vi "algoritmo_9.vi"() -> ()   [LabVIEW 2024]
uses:
  <vilib>/Platform/TimedLoop/XDataNode/timing_clust.ctl
  <vilib>/Platform/TimedLoop/XDataNode/nitl_modes.ctl
  <vilib>/Platform/TimedLoop/XDataNode/wakeup.ctl
  <vilib>/MakerHub/LINX/Public/Peripherals/PWM/PWM Set Duty Cycle 1 Chan.vi
  <vilib>/MakerHub/LINX/Public/Utilities/Open Serial.vi
  <vilib>/MakerHub/LINX/Public/Peripherals/PWM/PWM Set Duty Cycle N Chans.vi
  <vilib>/platform/TimedLoop/XDataNode/XDataNode.xnode
  <vilib>/Platform/TimedLoop/XDataNode/XDNodeRunTimeDep.lvlib
  <vilib>/MakerHub/LINX/LMH-LINX.lvlib
  <vilib>/MakerHub/LINX/Public/Sensors/Distance/Ultrasonic/Ultrasonic.lvlib
  <vilib>/Analysis/NI_AALPro.lvlib
panel:
  out "normal":dbl
  out "Integral":dbl
  out "poli":dbl
  out "pol":dbl
  in  "ESTIMAR":dbl(slide) scale=-41.0..41.0
  in  "Ref":dbl(slide) scale=5.0..41.0
  in  "POL":dbl(slide) scale=0.5..0.9
  in  "POLI":dbl(slide) scale=0.0..0.1
  in  "CONTROL":dbl
  out "Error":dbl
  out "PWM":dbl format="%0.2f"
  out "uk":dbl
  out "ESTADO":dbl
  out "MINUTOS":dbl format="%#_2g"
  out "Y_e":dbl
  out "error de estimacion":dbl
  out "THETA":cdb[](array[numeric])
  out "Waveform Chart":T1(graph)
  in  "stop":bool
  in  "Serial Port":refnum<visa-resource-name>="N/A"
  out "Error Out":errorcluster
  out "Y_Real":fxp<+/-,64,32>
  # "0 PARA ESTIMAR\n1 PARA CONTROLAR"
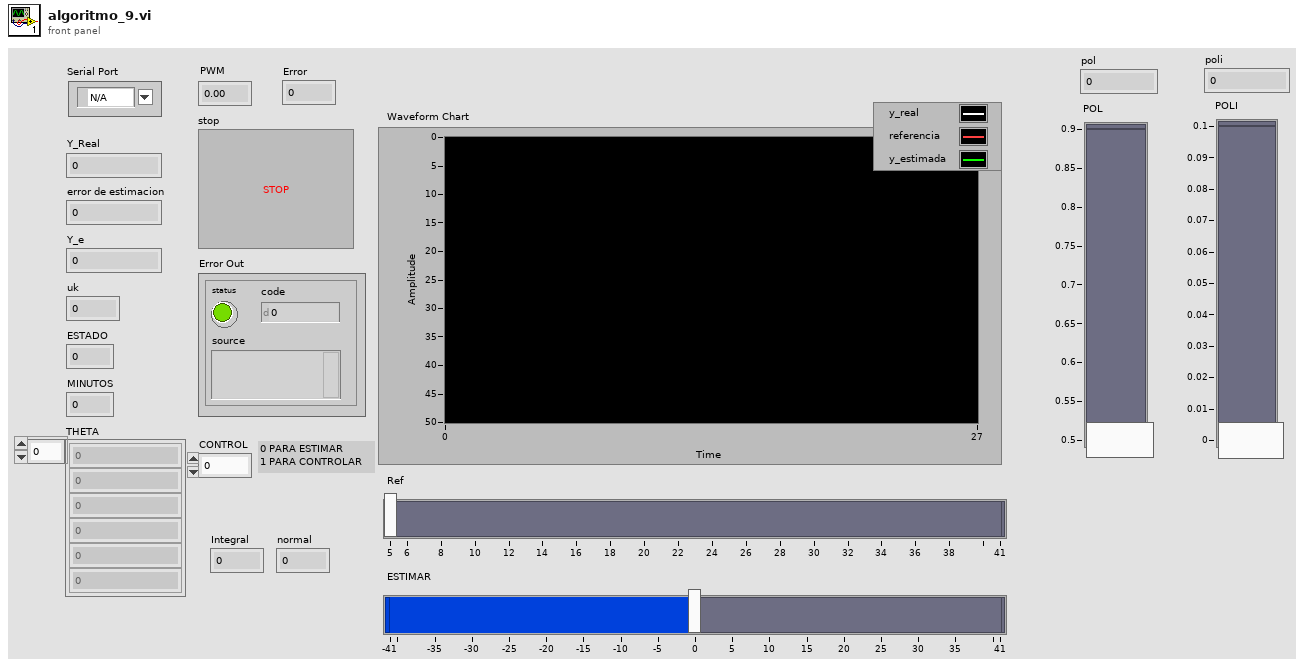
[diagram p1: front panel]
types:
  T1 = cluster{"Centimeters":dbl, "Referencia":dbl, dbl}
  T2 = typedef "LMH-LINX.lvlib/LINX Ref.ctl" = cluster{"IO":T3, "Interface":T4, "LINX Device Config":T5}
  T3 = typedef "LMH-LINX.lvlib/Platform.ctl" = enum16{"Remote", "Local"}
  T4 = typedef "LMH-LINX.lvlib/Interface.ctl" = enum16{"Serial", "TCP"}
  T5 = typedef "LMH-LINX.lvlib/Device.lvlib/LINX Device Config.ctl" = cluster{"Interface":T4, "COM Port":refnum<visa-resource-name>, "TCP Configuration":T6, "Device Family":u8, "Device ID":u8, "Device Name":string, "TCP Ref":refnum<k5>, "Channels":T7}
  T6 = typedef "LMH-LINX.lvlib/Device.lvlib/TCP Config.ctl" = cluster{"IP Address":string, "Port":u16}
  T7 = typedef "LMH-LINX.lvlib/Channels.ctl" = cluster{"DI":u8[], "DO":u8[], "AI":u8[], "AO":u8[], "PWM":u8[], "QE":u8[], "UART":u8[], "I2C 2":u8[], "SPI":u8[], "CAN":u8[], "Servo":u8[], "AI Ref (V)":dbl, "AI Resolution (Bits)":u8, "AO Ref (V)":dbl, "AO Resolution (Bits)":u8}
  T8 = typedef "XDNodeRunTimeDep.lvlib/timing_clust.ctl" = cluster{"Expected End [f-1]":u64, "Actual End [f-1]":u64, "Finished Late? [f-1]":bool, "Expected End [i-1]":u64, "Actual End [i-1]":u64, "Finished Late? [i-1]":bool, "Expected Start [i]":u64, "Actual Start [i]":u64, "Expected Start [f]":u64, "Actual Start [f]":u64, "Source Name":string, "Structure Name":string, "Period":i64, "Deadline":i64, "Offset":i64, "Start":i64, "Priority":i32, "Timeout":i32, "Mode":T9, "Wakeup Reason":T10, "Error":errorcluster, "Source Type":string, "Secondary Source Type":string, "Global End Time":u64, "Global Start Time":u64, "Frame Duration":u64, "Iteration Duration":u64, "Assigned CPU":i32, "I/O Scan Engine Mode":u32}
  T9 = typedef "XDNodeRunTimeDep.lvlib/nitl_modes.ctl" = enum32{"No Change", "Process missed periods, maintain original phase", "Discard missed periods, maintain original phase", "Process missed periods, ignore original phase", "Discard missed periods, ignore original phase"}
  T10 = typedef "XDNodeRunTimeDep.lvlib/wakeup.ctl" = enum32{"Normal", "Aborted", "Asynchronous wakeup", "Timing source error", "Timed loop error", "Timeout"}
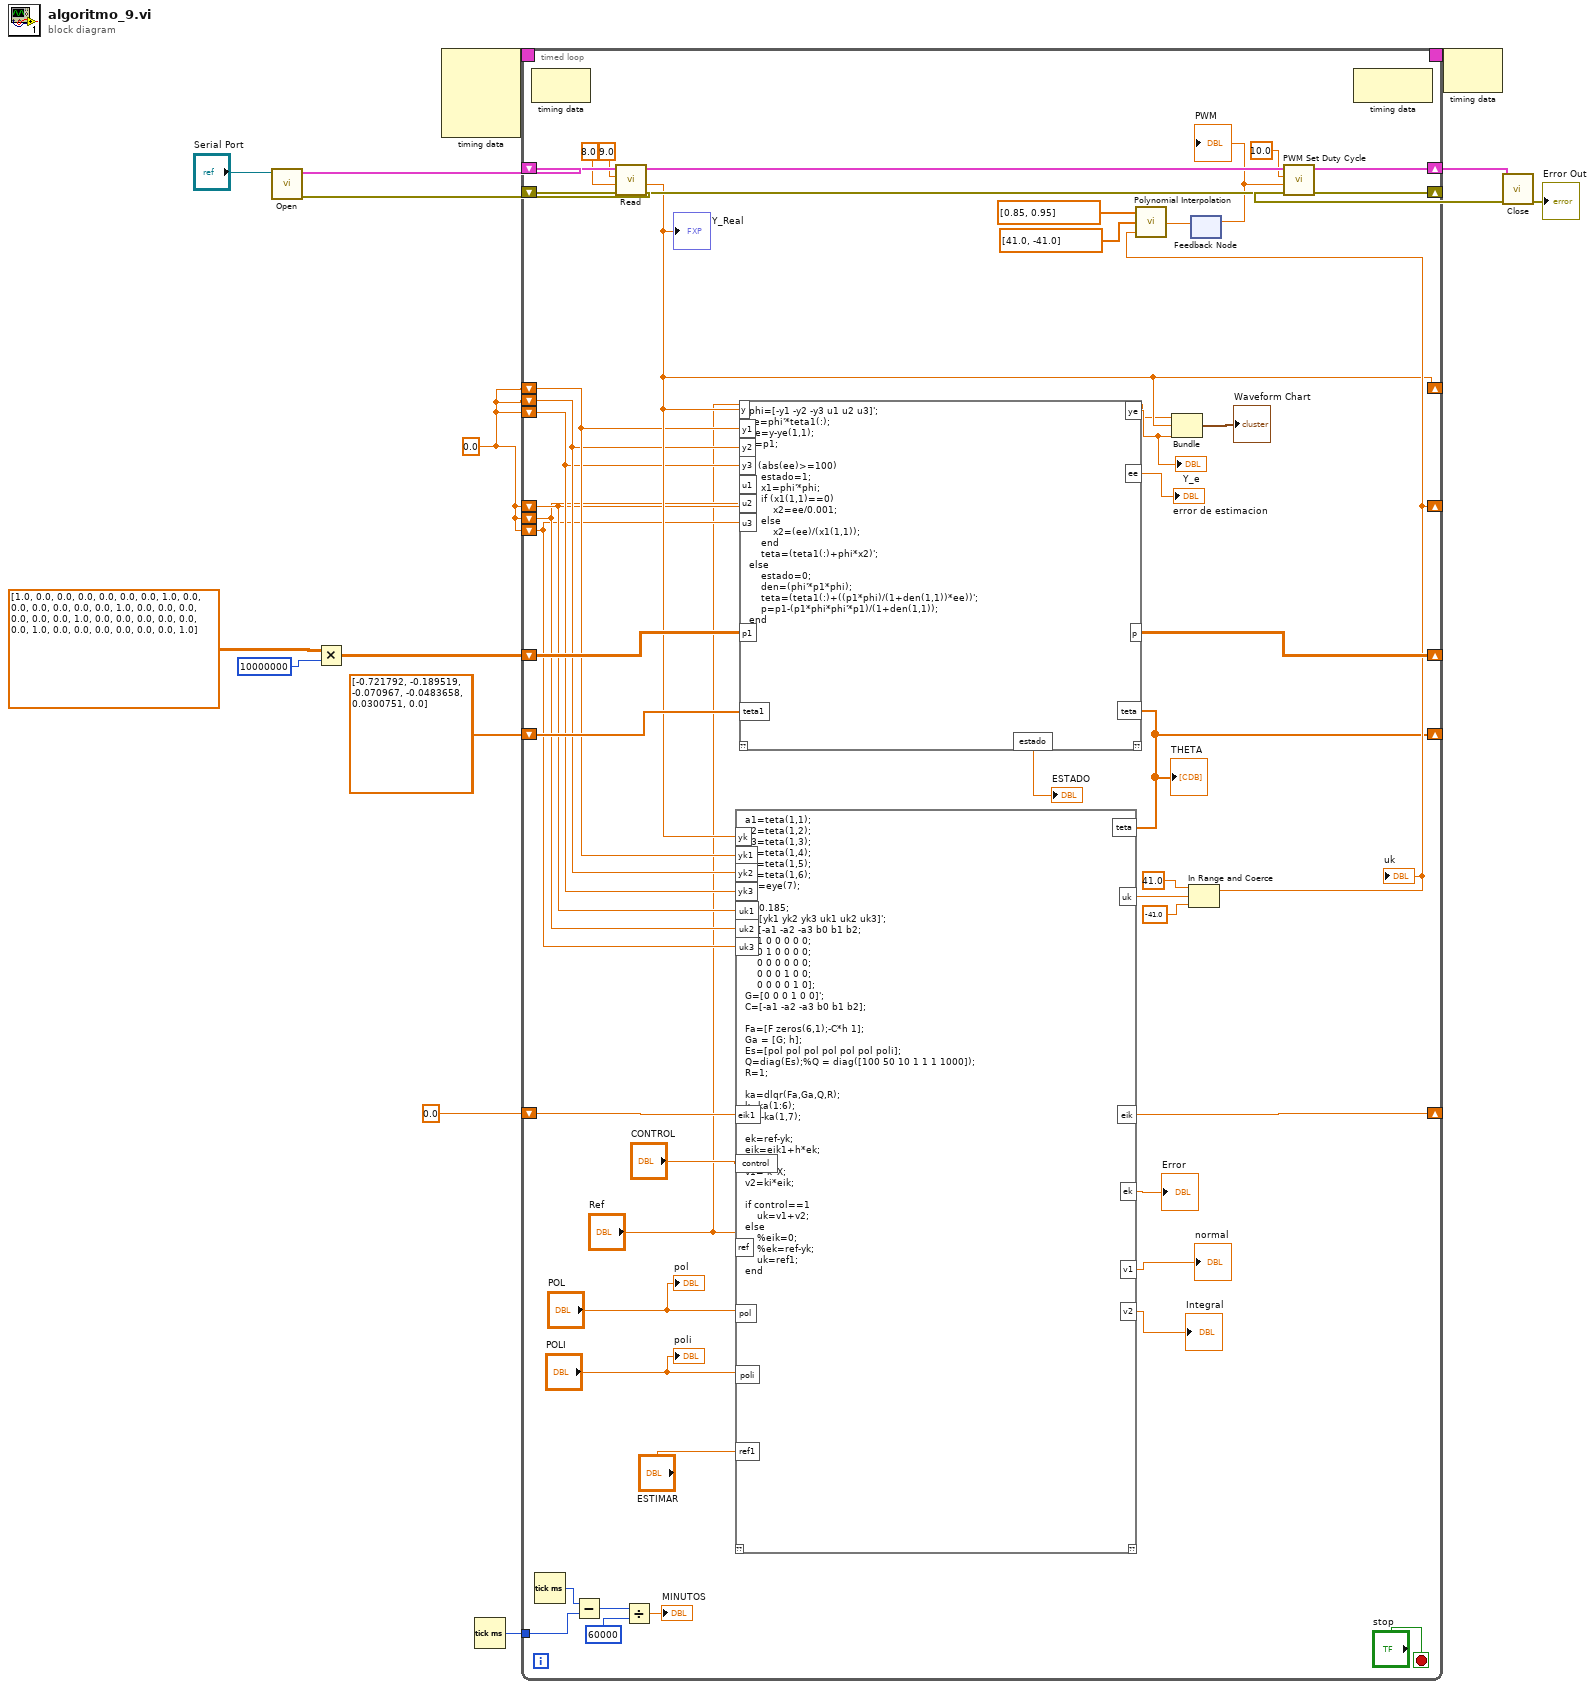
[diagram p0: block diagram]
diagram:
  (unwired) dbl[] [-0.721792, -0.189519, -0.070967, -0.0483658, 0.0300751, 0.0]
  w1 = 0.0
  n1 = call-poly <vilib>:"Open.vi"("Serial Port"="Serial Port") -> ("Error Out"=w11:errorcluster, "LINX Resource"=w13:T2)  [unwired: 8 in, 1 out]
  n2 = Multiply(x=dbl[][] [[1.0, 0.0, 0.0, 0.0, 0.0, 0.0], [0.0, 1.0, 0.0, 0.0, 0.0, 0.0], [0.0, 0.0, 1.0, 0.0, 0.0, 0.0], [0.0, 0.0, 0.0, 1.0, 0.0, 0.0], [0.0, 0.0, 0.0, 0.0, 1.0, 0.0], [0.0, 0.0, 0.0, 0.0, 0.0, 1.0]], y=10000000) -> (x*y=w5:dbl[][])
  n3 = node-c288() -> (w15:T8)  [unwired: 4 in]
  n4 = Tick Count (ms)() -> (millisecond timer value=w4:u32)
  n5 = timed-loop {
    timing: w15 -> [_]
    timing-out: [_] -> w14
    shift-right: [w52] -> w12
    shift-left: w13 -> [w63]
    shift-right: [w57] -> w10
    shift-left: w11 -> [w62]
    shift-right: [w23] -> _
    shift-left: dbl[] [-0.94337, -0.103907, 0.033856, -0.0056629, 0.00349643, 0.0144388] -> [w51]
    shift-right: [w30] -> _
    shift-left: w1 -> [w29]
    shift-right: [w31] -> _
    shift-left: w1 -> [w26]
    shift-left: w1 -> [w28]
    shift-left: w1 -> [w27]
    shift-left: w1 -> [w25]
    shift-left: w1 -> [w24]
    shift-right: [w48] -> _
    shift-left: w5 -> [w49]
    tunnel: w4 -> [w45]
    shift-right: [w37] -> _
    shift-left: 0.0 -> [w36]
    stop <- "stop" stop-if-true
    n6 = node-c288() -> ()  [unwired: 1 in, 1 out]
    n7 = Tick Count (ms)() -> (millisecond timer value=w46:u32)
    n8 = Subtract(x=w46, y=w45) -> (x-y=w43:u32)
    n9 = call <vilib>:"Read.vi"("Error In"=w62, "DO Channel"=8.0, "DI Channel"=9.0, "LINX Resource"=w63) -> ("Error Out"=w58:errorcluster, "Centimeters"=w30:dbl, "LINX Resource"=w59:T2)  [unwired: 4 in, 1 out]
    "Y_Real" <- w30
    n10 = Divide(x=w43, y=u32 60000) -> (x/y=→"MINUTOS":dbl)
    n11 = script code="phi=[-y1 -y2 -y3 u1 u2 u3]';\nye=phi'*teta1(:);\nee=y-ye(1,1);\np=p1;\n\nif (abs(ee)>=100)\n    estado=1;\n    x1=phi'*phi;\n    if (x1(1,1)==0)\n        x2=ee/0.001;\n    else\n        x2=(ee)/(x1(1,1));\n    end\n    teta=(teta1(:)+phi*x2)';\nelse\n    estado=0;\n    den=(phi'*p1*phi);\n    teta=(teta1(:)+((p1*phi)/(1+den(1,1))*ee))';\n    p=p1-(p1*phi*phi'*p1)/(1+den(1,1));\nend"("teta1"=w51, "y1"=w29, "y2"=w28, "y3"=w27, "u1"=w26, "u2"=w25, "u3"=w24, "y"=w30, "p1"=w49) -> ("teta"=w23:dbl[], "p"=w48:dbl[][], "ye"=w22:dbl, "ee"=→"error de estimacion":dbl, "estado"=→"ESTADO":dbl)  [unwired: 1 in, 1 out]
    "THETA" <- w23
    "Y_e" <- w22
    n12 = script code="a1=teta(1,1);\na2=teta(1,2);\na3=teta(1,3);\nb0=teta(1,4);\nb1=teta(1,5);\nb2=teta(1,6);\nQ1=eye(7);\n\nh=0.185;\nX=[yk1 yk2 yk3 uk1 uk2 uk3]';\nF=[-a1 -a2 -a3 b0 b1 b2;\n    1 0 0 0 0 0;\n    0 1 0 0 0 0;\n    0 0 0 0 0 0;\n    0 0 0 1 0 0;\n    0 0 0 0 1 0];\nG=[0 0 0 1 0 0]';\nC=[-a1 -a2 -a3 b0 b1 b2];\n\nFa=[F zeros(6,1);-C*h 1];\nGa = [G; h];\nEs=[pol pol pol pol pol pol poli];\nQ=diag(Es);%Q = diag([100 50 10 1 1 1 1000]);\nR=1;\n\nka=dlqr(Fa,Ga,Q,R);\nk=ka(1:6);\nki=-ka(1,7);\n\nek=ref-yk;\neik=eik1+h*ek;\n\nv1=-k*X;\nv2=ki*eik;\n\nif control==1\n    uk=v1+v2;\nelse\n    %eik=0;\n    %ek=ref-yk;\n    uk=ref1;\nend"("teta"=w23, "yk"=w30, "eik1"=w36, "control"="CONTROL", "ref"="Ref", "yk1"=w29, "yk2"=w28, "yk3"=w27, "uk1"=w26, "uk2"=w25, "uk3"=w24, "pol"="POL", "poli"="POLI", "ref1"="ESTIMAR") -> ("uk"=w38:dbl, "eik"=w37:dbl, "ek"=→"Error":dbl, "v1"=→"normal":dbl, "v2"=→"Integral":dbl)  [unwired: 1 in, 1 out]
    n13 = Bundle("Ref"="Ref", "Centimeters"=w30, w22) -> (→"Waveform Chart":cluster{"Ref ":dbl, "Centimeters":dbl, dbl})  [unwired: 1 in]
    n14 = In Range and Coerce(upper limit=41.0, x=w38, lower limit=-41.0) -> (coerced(x)=w31:dbl)  [unwired: 1 out]
    "uk" <- w31
    n15 = call <vilib>:"Polynomial Interpolation.vi"("x value"=w31, "X"=dbl[] [41.0, -41.0], "Y"=dbl[] [0.85, 0.95]) -> ("interpolation value"=w33:dbl)  [unwired: 2 out]
    n16 = feedback-in #1(w33) -> ()
    n17 = feedback #1() -> (w32:dbl)  [unwired: 1 in]
    "PWM" <- w32
    n18 = call-poly <vilib>:"PWM Set Duty Cycle.vi"("Error In"=w58, "Duty Cycle (0-1)"=w32, "PWM Channel"=10.0, "LINX Resource"=w59) -> ("Error Out"=w57:errorcluster, "LINX Resource"=w52:T2)  [unwired: 6 in]
    n19 = node-c288() -> ()  [unwired: 1 in, 1 out]
    "pol" <- "POL"
    "poli" <- "POLI"
  }
  n20 = node-c288(w14) -> ()  [unwired: 1 out]
  n21 = call <vilib>:"Close.vi"("Error In"=w10, "LINX Resource"=w12) -> ("Error Out"=→"Error Out":errorcluster)  [unwired: 9 in]
